vi "1D to 2D Array.vi"(10 "1D Array":dbl[](array[numeric]) format="%#_3g") -> (2 "2D Array":dbl[][](array[numeric]) format="%#_3g")   [LabVIEW 2013]
panel:
  in  "init array":dbl[][](array[numeric])=[[0.0, 0.0], [0.0, 0.0]]
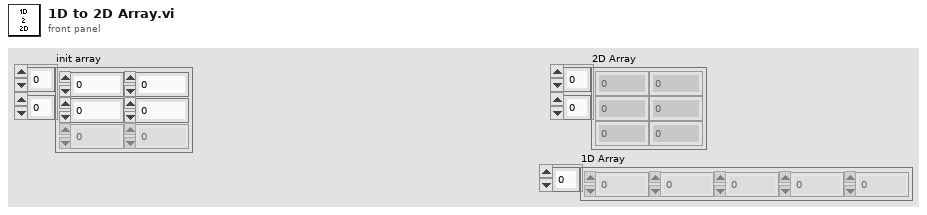
[diagram p1: front panel]
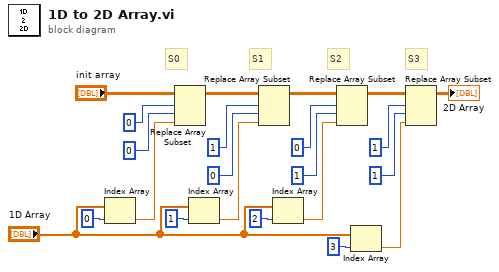
[diagram p0: block diagram]
diagram:
  # "S3"
  # "S2"
  # "S1"
  # "S0"
  n1 = Index Array(array="1D Array", index=0) -> (element=w5:dbl)
  n2 = Replace Array Subset(array="init array", new element=w5, index (row)=0, index (col)=0 ("disabled index (col)")) -> (w15:dbl[][])
  n3 = Index Array(array="1D Array", index=1) -> (element=w4:dbl)
  n4 = Replace Array Subset(array=w15, new element=w4, index (row)=1, index (col)=0 ("disabled index (col)")) -> (w14:dbl[][])
  n5 = Index Array(array="1D Array", index=2) -> (element=w3:dbl)
  n6 = Replace Array Subset(array=w14, new element=w3, index (row)=0, index (col)=1 ("disabled index (col)")) -> (w13:dbl[][])
  n7 = Index Array(array="1D Array", index=3) -> (element=w2:dbl)
  n8 = Replace Array Subset(array=w13, new element=w2, index (row)=1, index (col)=1 ("disabled index (col)")) -> (→"2D Array":dbl[][])
